vi "BuildPacket.vi"(1 "Counter":i16, 2 "Dummy":i16) -> (0 "PacketArray":i32[](array[numeric]))   [LabVIEW 2010]
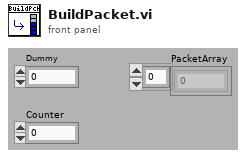
[diagram p1: front panel]
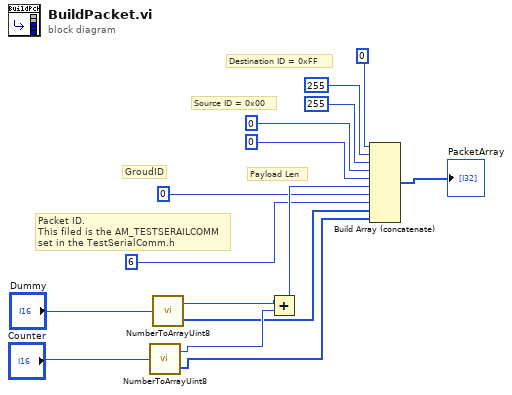
[diagram p0: block diagram]
diagram:
  # "Packet ID.\nThis filed is the AM_TESTSERAILCOMM \nset in the TestSerialComm.h"
  # "GroudID"
  # "Payload Len"
  # "Source ID = 0x00"
  # "Destination ID = 0xFF"
  n1 = call "NumberToArrayUint8.vi"("Numeric 2"="Counter") -> ("Array"=w10:i8[], "Numeric"=w13:i32)
  n2 = call "NumberToArrayUint8.vi"("Numeric 2"="Dummy") -> ("Array"=w8:i8[], "Numeric"=w11:i32)
  n3 = Add(x=w11, y=w13) -> (x+y=w12:i32)
  n4 = Build Array (concatenate)(0, 255, 255, 0, 0, w12, 0, i8 6, w8, w10) -> (→"PacketArray":i32[])
